vi "Actor Core.vi"(8 "error in":errorcluster, 11 "Nested in":refnum<class "LaserController.lvclass">) -> (0 "error out":errorcluster, 3 "Actor out":refnum<class "Actor.lvclass">)   [LabVIEW 2020, in "LaserController.lvlib" / "LaserController.lvclass"]
doc: "(<B>Filename</B>: Actor Framework.lvlib:Actor.lvclass:Actor Core.vi)\n\nReceives messages to the actor, reacts to them, and initiates any error handling that may shut the actor down.\n\nDescendant classes may override this VI to append parallel tasks for the actor to complete while it handles messages. Overrides use the Call Parent Method node."
uses:
  LaserController.lvclass
  <vilib>/ActorFramework/Actor/Actor.lvclass
  <vilib>/ActorFramework/Stop Msg/Stop Msg.lvclass
  Model/Hardware Abstraction Layer/Component/Laser/Laser Messages/SetPower Msg/SetPower Msg.lvclass
  Model/Hardware Abstraction Layer/Component/Laser/Laser Messages/GetPower Msg/GetPower Msg.lvclass
  Model/Hardware Abstraction Layer/Component/Laser/Laser Messages/SetShutterStatus Msg/SetShutterStatus Msg.lvclass
  Model/Hardware Abstraction Layer/Component/Laser/Laser Messages/SetAutoShutter Msg/SetAutoShutter Msg.lvclass
  Model/Hardware Abstraction Layer/Component/GenericActor/GenericActor/GenericController.lvclass
  E:/Development/DevHardSoftware/MicroscopyFramework/Model/Hardware Abstraction Layer/Component/GenericActor/GenericActor/GenericController.lvclass
  C:/Program Files/National Instruments/LabVIEW 2020/vi.lib/ActorFramework/Actor/Actor.lvclass
  E:/Development/DevHardSoftware/MicroscopyFramework/Interface/DataGenerator/DataGenerator.lvclass
  E:/Development/DevHardSoftware/MicroscopyFramework/Interface/DataListener/DataListener.lvclass
  E:/Development/DevHardSoftware/MicroscopyFramework/Interface/ErrorHandler/ErrorHandler.lvclass
  E:/Development/DevHardSoftware/MicroscopyFramework/ViewController/OxxiusLaserController/LaserController.lvclass
panel:
  in  "405 Auto":bool caption="LAS-05997"
  in  "488 Auto":bool caption="LAS-06030"
  in  "532 Auto":bool caption="LAS-05886"
  in  "561 Auto":bool caption="LAS-05858"
  in  "647 Auto":bool caption="LAS-05914"
  in  "785 Auto":bool caption="LAS-03914"
  in  "785 Power":sgl caption="LAS-03914" min=0 max=200
  in  "785/50mW":bool caption="LAS-03914"
  in  "647 Power":sgl caption="LAS-05914"
  in  "647/140mW":bool caption="LAS-05914"
  in  "561 Power":sgl caption="LAS-05858" min=0 max=200
  in  "561/100mW":bool caption="LAS-05858"
  in  "532 Power":sgl caption="LAS-05886" min=0 max=200
  in  "532/100mW":bool caption="LAS-05886"
  in  "488 Power":sgl caption="LAS-06030" min=0 max=200
  in  "488/150mW":bool caption="LAS-06030"
  in  "405 Power":sgl caption="LAS-05997" min=0 max=200
  in  "405/180mW":bool caption="LAS-05997"
  # "Power(%)"
  # "On/Off"
  # "AutoShutter"
  # "Lasers"
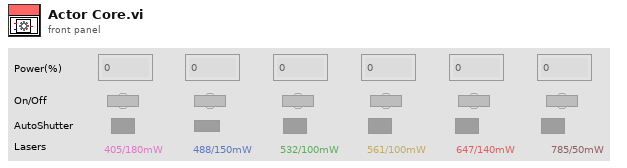
[diagram p1: front panel]
types:
  T1 = cluster{"Status":refnum<vi>, "Auto":refnum<vi>, "Power":refnum<vi>}
  T2 = map{string, cluster{"Status":refnum<vi>, "Auto":refnum<vi>, "Power":refnum<vi>}}
  T3 = cluster{"Stop":refnum<user-event>, "Visible":refnum<user-event>, "Update Power":refnum<user-event>}
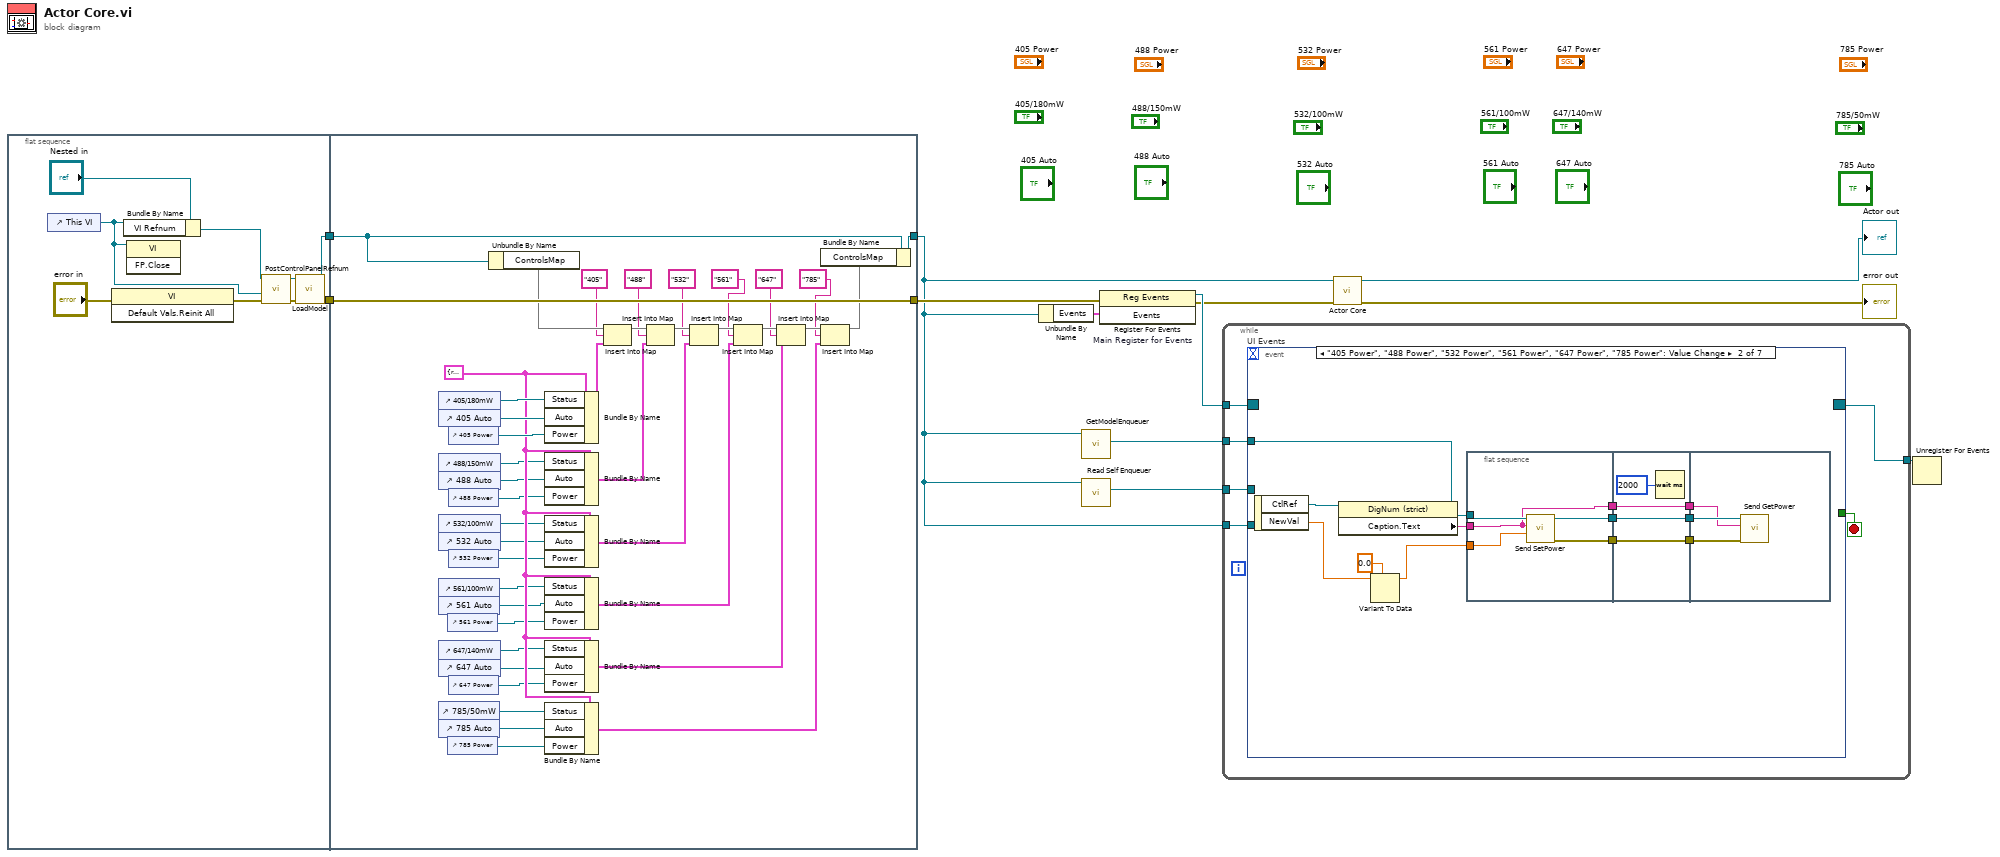
[diagram p0: block diagram]
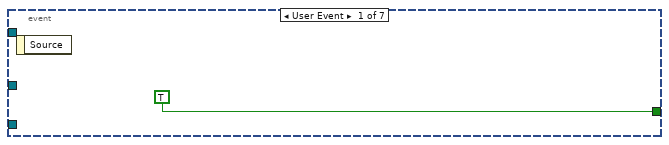
[diagram p2: hidden frame]
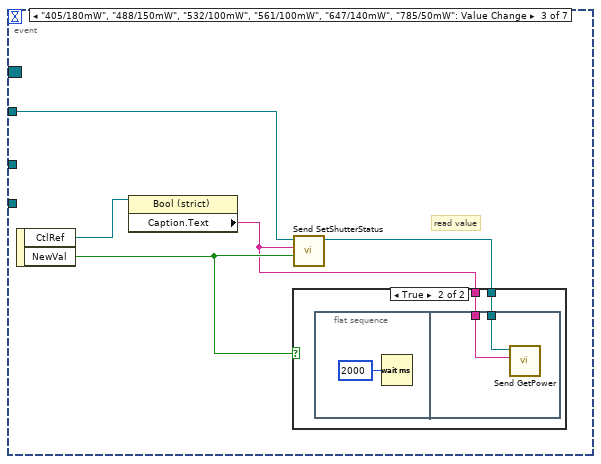
[diagram p3: hidden frame]
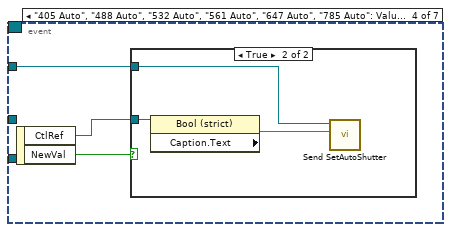
[diagram p5: hidden frame]
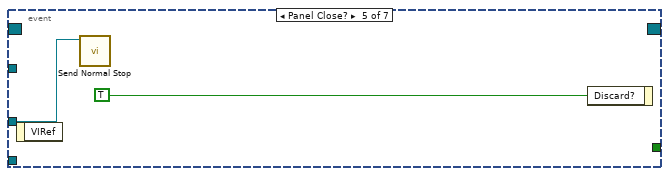
[diagram p7: hidden frame]
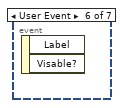
[diagram p8: hidden frame]
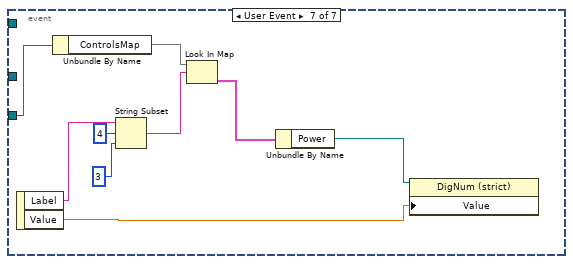
[diagram p9: hidden frame]
diagram:
  n1 = flat-sequence {
    tunnel: [w15] -> w4
    tunnel: [w13] -> w3
    tunnel: [w61] -> w1
    tunnel: [w62] -> w5
    tunnel: w4 -> [w62]
    tunnel: w3 -> [w60]
    frame #0 {
      n2 = control-ref of="This VI"() -> (w16:refnum<vi>)
      n3 = invoke class="VI" method="Default Vals.Reinit All"(error in="error in") -> (error out=w19:errorcluster)  [unwired: 2 in, 2 out]
      n4 = Bundle By Name(cluster="Nested in", "VI Refnum"=w16) -> (w17:refnum<class "LaserController.lvclass">)
      n5 = invoke class="VI" method="FP.Close"(reference=w16) -> ()  [unwired: 2 in, 3 out]
      n6 = call-dynamic "PostControlPanelRefnum.vi"("error in (no error)"=w19, "VI Refnum"=w16, "GRMActor in"=w17) -> ("error out"=w18:errorcluster, "GRMActor out"=w14:refnum<class "LaserController.lvclass">)  [unwired: 7 in]
      n7 = call-dynamic "LoadModel.vi"("error in (no error)"=w18, "GRMActor in"=w14) -> ("error out"=w15:errorcluster, "GRMActor out"=w13:refnum<class "LaserController.lvclass">)  [unwired: 8 in]
    }
    frame #1 {
      w53 = T1 {"Status"=refnum, "Auto"=refnum, "Power"=refnum} ("value")
      n8 = control-ref of="561/100mW"() -> (w30:refnum<vi>)
      n9 = control-ref of="561 Auto"() -> (w29:refnum<vi>)
      n10 = control-ref of="785/50mW"() -> (w24:refnum<vi>)
      n11 = control-ref of="785 Auto"() -> (w23:refnum<vi>)
      n12 = control-ref of="405/180mW"() -> (w56:refnum<vi>)
      n13 = control-ref of="405 Auto"() -> (w55:refnum<vi>)
      n14 = control-ref of="488/150mW"() -> (w31:refnum<vi>)
      n15 = control-ref of="488 Auto"() -> (w32:refnum<vi>)
      n16 = control-ref of="532/100mW"() -> (w36:refnum<vi>)
      n17 = control-ref of="532 Auto"() -> (w35:refnum<vi>)
      n18 = control-ref of="647/140mW"() -> (w27:refnum<vi>)
      n19 = control-ref of="647 Auto"() -> (w26:refnum<vi>)
      n20 = control-ref of="561 Power"() -> (w28:refnum<vi>)
      n21 = control-ref of="785 Power"() -> (w22:refnum<vi>)
      n22 = control-ref of="405 Power"() -> (w54:refnum<vi>)
      n23 = control-ref of="488 Power"() -> (w33:refnum<vi>)
      n24 = control-ref of="532 Power"() -> (w34:refnum<vi>)
      n25 = control-ref of="647 Power"() -> (w25:refnum<vi>)
      n26 = Unbundle By Name(w60) -> ("ControlsMap"=w59:T2)
      n27 = Bundle By Name(cluster=w53, "Status"=w56, "Auto"=w55, "Power"=w54) -> (w57:T1)
      n28 = Bundle By Name(cluster=w53, "Status"=w31, "Auto"=w32, "Power"=w33) -> (w41:T1)
      n29 = Bundle By Name(cluster=w53, "Status"=w36, "Auto"=w35, "Power"=w34) -> (w40:T1)
      n30 = Bundle By Name(cluster=w53, "Status"=w30, "Auto"=w29, "Power"=w28) -> (w39:T1)
      n31 = Bundle By Name(cluster=w53, "Status"=w27, "Auto"=w26, "Power"=w25) -> (w38:T1)
      n32 = Bundle By Name(cluster=w53, "Status"=w24, "Auto"=w23, "Power"=w22) -> (w37:T1)
      n33 = Insert Into Map(map in=w59, key="405", value=w57) -> (map out=w52:T2)  [unwired: 2 out]
      n34 = Insert Into Map(map in=w52, key="488", value=w41) -> (map out=w51:T2)  [unwired: 2 out]
      n35 = Insert Into Map(map in=w51, key="532", value=w40) -> (map out=w50:T2)  [unwired: 2 out]
      n36 = Insert Into Map(map in=w50, key="561", value=w39) -> (map out=w49:T2)  [unwired: 2 out]
      n37 = Insert Into Map(map in=w49, key="647", value=w38) -> (map out=w48:T2)  [unwired: 2 out]
      n38 = Insert Into Map(map in=w48, key="785", value=w37) -> (map out=w47:T2)  [unwired: 2 out]
      n39 = Bundle By Name(cluster=w60, "ControlsMap"=w47) -> (w61:refnum<class "LaserController.lvclass">)
    }
  }
  n40 = Unbundle By Name(w1) -> ("Events"=w9:T3)
  n41 = call-dynamic "GetModelEnqueuer.vi"("GRMActor in"=w1) -> ("ModelEnqueuer"=w2:refnum<class "Message Enqueuer.lvclass">)  [unwired: 8 in, 2 out]
  n42 = call <vilib>:"Read Self Enqueuer.vi"("Actor"=w1) -> ("Self Enqueuer"=w7:refnum<class "Message Enqueuer.lvclass">)  [unwired: 10 in]
  n43 = register-events "Main Register for Events"(error in=w5, w9) -> (reference out=w10:refnum<event-registration>, error out=w6:errorcluster)  [unwired: 1 in]
  n44 = while {
    tunnel: w10 -> [w68]
    tunnel: [w66] -> w8
    tunnel: w7 -> [w65]
    tunnel: w2 -> [w64]
    tunnel: w1 -> [w63]
    stop <- w67 stop-if-true
    n45 = event "UI Events" shown="[1] \"405 Power\", \"488 Power\", \"532 Power\", \"561 Power\", \"647 Power\", \"785 Power\": Value Change" {
      selector: w68 -> [_ _ _ _ _ _ _]
      dyn-events: [_ _ _ _ _ _ _] -> w66
      timeout: _ -> [_ _ _ _ _ _ _]
      tunnel: [TRUE _ _ _ _ _ _] -> w67
      tunnel: w65 -> [_ _ _ _ w110 _ _]
      tunnel: w64 -> [_ w76 w98 w106 _ _ _]
      tunnel: w63 -> [_ _ _ _ _ _ w116]
      event User Event {
        n46 = event-data() -> ()  [unwired: 1 in, 1 out]
      }
      event "405 Power", "488 Power", "532 Power", "561 Power", "647 Power", "785 Power": Value Change {
        n47 = event-data() -> ("CtlRef"=w81:refnum<vi>, "NewVal"=w80:sgl)  [unwired: 1 in]
        n48 = property class="DigNum (strict)"(reference=w81) -> ("Caption.Text"=w77:string)  [unwired: 1 in, 2 out]
        n49 = Variant To Data(type=0.0 ("Value"), Variant=w80) -> (data=w78:dbl)  [unwired: 1 in, 1 out]
        n50 = flat-sequence {
          tunnel: w78 -> [w86]
          tunnel: w77 -> [w82]
          tunnel: w76 -> [w85]
          tunnel: [w84] -> w75
          tunnel: [w83] -> w73
          tunnel: [w82] -> w71
          tunnel: w75 -> [w90]
          tunnel: [w90] -> w74
          tunnel: w73 -> [w89]
          tunnel: [w89] -> w72
          tunnel: w71 -> [w88]
          tunnel: [w88] -> w70
          tunnel: w74 -> [w93]
          tunnel: w72 -> [w92]
          tunnel: w70 -> [w91]
          frame #0 {
            n51 = call "Send SetPower.vi"("Value"=w86, "Label"=w82, "Message Enqueuer"=w85) -> ("error out"=w84:errorcluster, "Message Enqueuer out"=w83:refnum<class "Message Enqueuer.lvclass">)  [unwired: 7 in]
          }
          frame #1 {
            n52 = Wait (ms)(milliseconds to wait=u32 2000) -> ()  [unwired: 1 out]
          }
          frame #2 {
            n53 = call "Send GetPower.vi"("error in (no error)"=w93, "Label"=w91, "Message Enqueuer"=w92) -> ()  [unwired: 7 in, 2 out]
          }
        }
      }
      event "405/180mW", "488/150mW", "532/100mW", "561/100mW", "647/140mW", "785/50mW": Value Change {
        # "read value"
        n54 = event-data() -> ("CtlRef"=w97:refnum<vi>, "NewVal"=w96:bool)  [unwired: 1 in]
        n55 = property class="Bool (strict)"(reference=w97) -> ("Caption.Text"=w94:string)  [unwired: 1 in, 2 out]
        n56 = call "Send SetShutterStatus.vi"("Value"=w96, "Label"=w94, "Message Enqueuer"=w98) -> ("Message Enqueuer out"=w95:refnum<class "Message Enqueuer.lvclass">)  [unwired: 7 in, 1 out]
        n57 = case shown="True" w96 {
          tunnel: w95 -> [_ w100]
          tunnel: w94 -> [_ w99]
          frame False {
          }
          frame True {
            n58 = flat-sequence {
              tunnel: w100 -> [w103]
              tunnel: w99 -> [w102]
              frame #0 {
                n59 = Wait (ms)(milliseconds to wait=u32 2000) -> ()  [unwired: 1 out]
              }
              frame #1 {
                n60 = call "Send GetPower.vi"("Label"=w102, "Message Enqueuer"=w103) -> ()  [unwired: 8 in, 2 out]
              }
            }
          }
        }
      }
      event "405 Auto", "488 Auto", "532 Auto", "561 Auto", "647 Auto", "785 Auto": Value Change {
        n61 = event-data() -> ("CtlRef"=w105:refnum<vi>, "NewVal"=w104:bool)  [unwired: 1 in]
        n62 = case shown="True" w104 {
          tunnel: w106 -> [_ w109]
          tunnel: w105 -> [_ w108]
          frame False {
          }
          frame True {
            n63 = property class="Bool (strict)"(reference=w108) -> ("Caption.Text"=w107:string)  [unwired: 1 in, 2 out]
            n64 = call "Send SetAutoShutter.vi"("Label"=w107, "Message Enqueuer"=w109) -> ()  [unwired: 8 in, 2 out]
          }
        }
      }
      event Panel Close? {
        n65 = event-data() -> ()  [unwired: 1 in, 1 out]
        n66 = call <vilib>:"Send Normal Stop.vi"("Message Enqueuer"=w110) -> ()  [unwired: 10 in, 1 out]
        n67 = event-data("Discard?"=TRUE) -> ()  [unwired: 1 in, 1 out]
      }
      event User Event {
        n68 = event-data() -> ()  [unwired: 1 in, 2 out]
      }
      event User Event {
        n69 = event-data() -> ("Label"=w117:string, "Value"=w120:dbl)  [unwired: 1 in]
        n70 = Unbundle By Name(w116) -> ("ControlsMap"=w115:T2)
        n71 = String Subset(string=w117, offset (0)=4, length (rest)=3 ("length (rest)")) -> (substring=w114:string)
        n72 = Look In Map(map=w115, key=w114) -> (value=w113:T1)  [unwired: 1 in, 1 out]
        n73 = Unbundle By Name(w113) -> ("Power"=w112:refnum<vi>)
        n74 = property class="DigNum (strict)"(reference=w112, "Value"=w120) -> ()  [unwired: 1 in, 2 out]
      }
    }
  }
  n75 = call-parent "Actor Core.vi"("error in"=w6, "Actor in"=w1) -> ("error out"=→"error out":errorcluster, "Actor out"=→"Actor out":refnum<class "Actor.lvclass">)  [unwired: 8 in]
  n76 = Unregister For Events(event registration refnum=w8) -> ()  [unwired: 1 in, 1 out]
